vi "Process Executor Object--constant.vi"() -> (3 "Process Executor.lvclass":refnum<class "Process Executor.lvclass">)   [LabVIEW 2025]
doc: "Return an object of Process Executor.lvclass"
uses:
  Process Executor/Process Executor.lvclass
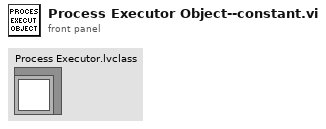
[diagram p1: front panel]
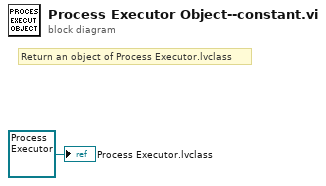
[diagram p0: block diagram]
diagram:
  # "Return an object of Process Executor.lvclass"
  "Process Executor.lvclass" <- refnum<class "Process Executor.lvclass"> refnum ("Process Executor.lvclass")
